vi "swerve_optimize_normalize.vi"(9 "Max Speed (m/s)":dbl, 11 "in ModuleStates":T1[](array[typedef]) {"Angle"."SIN" format="%13.4f"; "Angle"."COS" format="%13.4f"; "Angle"."VALUE" format="%13.4f"}) -> (3 "out ModuleStates":T1[](array[typedef]) {"Angle"."SIN" format="%13.4f"; "Angle"."COS" format="%13.4f"; "Angle"."VALUE" format="%13.4f"})   [LabVIEW 2020]
uses:
  <vilib>/Rock Robotics/WPI/ThirdParty/JAS_Junk/TrajLib/SWERVE_DRIVE_MODULE_STATE.ctl
  <vilib>/Rock Robotics/WPI/ThirdParty/JAS_Junk/TrajLib/ROTATION2D.ctl
  <vilib>/Rock Robotics/WPI/ThirdParty/JAS_Junk/TrajLib/Conv_Deg_Radians.vi
  <vilib>/Rock Robotics/WPI/ThirdParty/JAS_Junk/TrajLib/Rotation_CreateAngle.vi
  <vilib>/Rock Robotics/WPI/ThirdParty/JAS_Junk/TrajLib/Rotation_GetDegrees.vi
  <vilib>/Rock Robotics/WPI/ThirdParty/JAS_Junk/TrajLib/Units_RadiansToDegrees.vi
  <vilib>/Rock Robotics/WPI/ThirdParty/JAS_Junk/TrajLib/Rotation_GetRadians.vi
  <vilib>/Rock Robotics/WPI/ThirdParty/JAS_Junk/TrajLib/Conv_Radians_Deg.vi
  swerve_globals.vi
  swerve_best_angle.vi
  <vilib>/Rock Robotics/WPI/ThirdParty/JAS_Junk/TrajLib/Trajectory_Library.lvlib
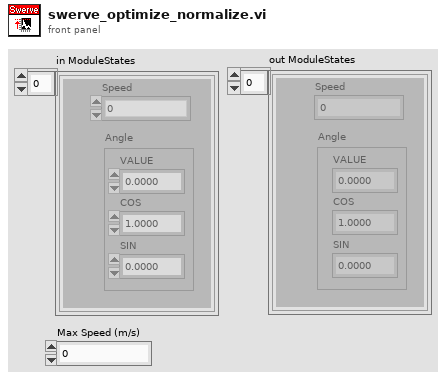
[diagram p1: front panel]
types:
  T1 = typedef "Trajectory_Library.lvlib/SWERVE_DRIVE_MODULE_STATE.ctl" = cluster{"Speed":dbl, "Angle":T2}
  T2 = typedef "Trajectory_Library.lvlib/ROTATION2D.ctl" = cluster{"VALUE":dbl, "COS":dbl, "SIN":dbl}
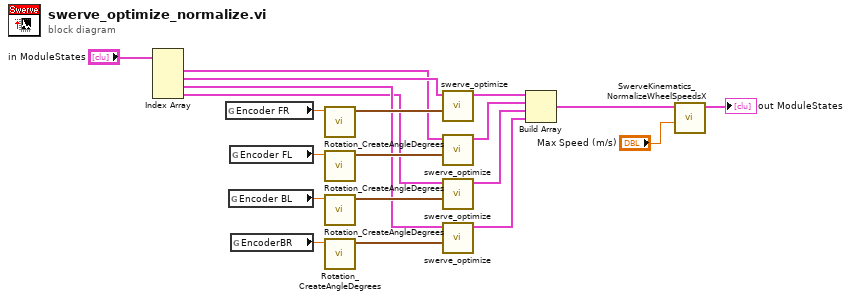
[diagram p0: block diagram]
diagram:
  n1 = Index Array(array="in ModuleStates") -> (element #1=w3:T1, element #2=w4:T1, element #3=w2:T1, element #4=w1:T1)  [unwired: 4 in]
  n2 = global read "swerve_globals.vi" "Encoder FR"() -> (w6:dbl)
  n3 = global read "swerve_globals.vi" "Encoder BL"() -> (w8:dbl)
  n4 = global read "swerve_globals.vi" "Encoder FL"() -> (w7:dbl)
  n5 = global read "swerve_globals.vi" "EncoderBR"() -> (w9:dbl)
  n6 = call <vilib>:"Rotation_CreateAngleDegrees.vi"("Angle_Degrees"=w6) -> ("ROTATION"=w13:T2)  [unwired: 10 in]
  n7 = call <vilib>:"Rotation_CreateAngleDegrees.vi"("Angle_Degrees"=w7) -> ("ROTATION"=w12:T2)  [unwired: 10 in]
  n8 = call <vilib>:"Rotation_CreateAngleDegrees.vi"("Angle_Degrees"=w8) -> ("ROTATION"=w11:T2)  [unwired: 10 in]
  n9 = call <vilib>:"Rotation_CreateAngleDegrees.vi"("Angle_Degrees"=w9) -> ("ROTATION"=w10:T2)  [unwired: 10 in]
  n10 = call "swerve_optimize.vi"("CurrentAngle"=w13, "Desired State"=w4) -> ("Output State"=w17:T1)  [unwired: 9 in]
  n11 = call "swerve_optimize.vi"("CurrentAngle"=w12, "Desired State"=w3) -> ("Output State"=w16:T1)  [unwired: 9 in]
  n12 = call "swerve_optimize.vi"("CurrentAngle"=w11, "Desired State"=w1) -> ("Output State"=w15:T1)  [unwired: 9 in]
  n13 = call "swerve_optimize.vi"("CurrentAngle"=w10, "Desired State"=w2) -> ("Output State"=w14:T1)  [unwired: 9 in]
  n14 = Build Array(w17, w16, w15, w14) -> (w18:T1[])
  n15 = call <vilib>:"SwerveKinematics_NormalizeWheelSpeedsX.vi"("AttainableMaxSpeed"="Max Speed (m/s)", "in WheelStates"=w18) -> ("out WheelStates"=→"out ModuleStates":T1[])  [unwired: 9 in]
